vi "AFM_Driver_Manager.Shutdown.vi"(8 "error in (no error)":errorcluster, 11 "AFM_Driver_Manager in":refnum<class "AFM_Driver_Manager.lvclass">) -> (0 "error out":errorcluster)   [LabVIEW 2019, in "AFM_Driver_Manager.lvclass"]
uses:
  AFM_Driver_Manager.lvclass
  AFM_Driver_Manager.lvclass/AFM_Driver_Manager.ctl
panel:
  out "AFM_Driver_Manager out":refnum<class "AFM_Driver_Manager.lvclass">
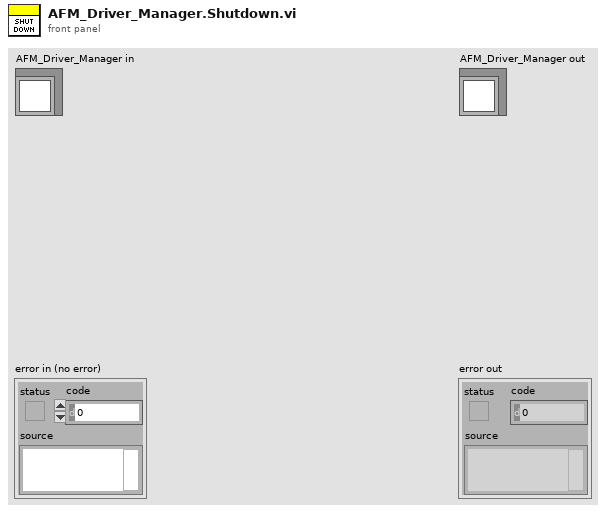
[diagram p1: front panel]
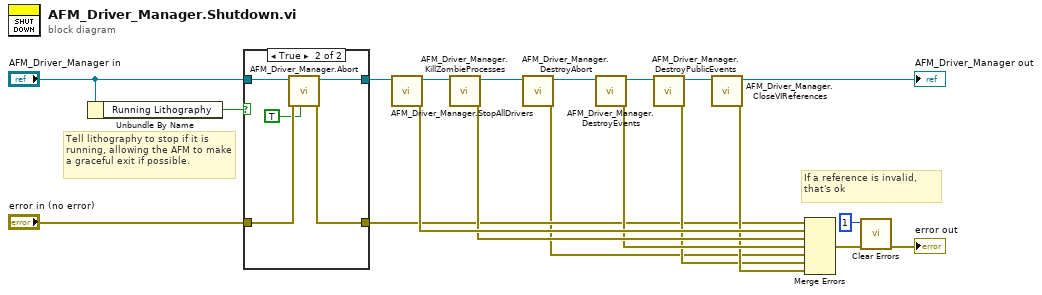
[diagram p0: block diagram]
diagram:
  # "Tell lithography to stop if it is running, allowing the AFM to make a graceful exit if possible."
  # "If a reference is invalid, that's ok"
  n1 = Unbundle By Name("AFM_Driver_Manager in") -> ("Running Lithography"=w7:bool)
  n2 = case shown="True" w7 {
    tunnel: "AFM_Driver_Manager in" -> [w22 w26]
    tunnel: [w22 w27] -> w8
    tunnel: "error in (no error)" -> [w21 w24]
    tunnel: [w21 w25] -> w5
    frame False {
    }
    frame True {
      n3 = call "AFM_Driver_Manager.Abort.vi"("Force? (F)"=TRUE, "error in (no error)"=w24, "AFM_Driver_Manager in"=w26) -> ("error out"=w25:errorcluster, "AFM_Driver_Manager out"=w27:refnum<class "AFM_Driver_Manager.lvclass">)  [unwired: 7 in]
    }
  }
  n4 = call "AFM_Driver_Manager.StopAllDrivers.vi"("AFM_Driver_Manager in"=w8) -> ("error out"=w20:errorcluster, "AFM_Driver_Manager out"=w18:refnum<class "AFM_Driver_Manager.lvclass">)  [unwired: 9 in]
  n5 = call "AFM_Driver_Manager.KillZombieProcesses.vi"("AFM_Driver_Manager in"=w18) -> ("error out"=w19:errorcluster, "AFM_Driver_Manager out"=w4:refnum<class "AFM_Driver_Manager.lvclass">)  [unwired: 9 in]
  n6 = call "AFM_Driver_Manager.DestroyAbort.vi"("AFM_Driver_Manager in"=w4) -> ("error out"=w2:errorcluster, "AFM_Driver_Manager out"=w3:refnum<class "AFM_Driver_Manager.lvclass">)  [unwired: 9 in]
  n7 = call "AFM_Driver_Manager.DestroyEvents.vi"("AFM_Driver_Manager in"=w3) -> ("error out"=w17:errorcluster, "AFM_Driver_Manager out"=w12:refnum<class "AFM_Driver_Manager.lvclass">)  [unwired: 9 in]
  n8 = call "AFM_Driver_Manager.DestroyPublicEvents.vi"("AFM_Driver_Manager in"=w12) -> ("error out"=w10:errorcluster, "AFM_Driver_Manager out"=w11:refnum<class "AFM_Driver_Manager.lvclass">)  [unwired: 9 in]
  n9 = call "AFM_Driver_Manager.CloseVIReferences.vi"("AFM_Driver_Manager in"=w11) -> ("error out"=w15:errorcluster, "AFM_Driver_Manager out"=→"AFM_Driver_Manager out":refnum<class "AFM_Driver_Manager.lvclass">)  [unwired: 9 in]
  n10 = Merge Errors(w5, w20, w19, w17, w2, w10, w15) -> (w9:errorcluster)
  n11 = call <vilib>:"Clear Errors.vi"("error in (no error)"=w9, "specific error code to clear (0: all)"=1) -> ("error out"=→"error out":errorcluster)  [unwired: 4 in, 1 out]
